vi "microflow_transducers.vi"   [LabVIEW 2017, in "sensor_translation.lvlib"]
uses:
  sensor_translation.lvlib
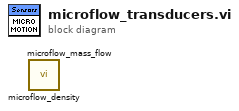
[diagram p0: block diagram]
diagram:
  n1 = call "microflow_density.vi"() -> ()  [unwired: 4 in, 1 out]
  n2 = call "microflow_mass_flow.vi"() -> ()  [unwired: 4 in, 1 out]
